vi "Read value Elevator Position.vi"(8 "error in (no error)":errorcluster, 11 "Sim Sensor Interface in":refnum<class "Sim Sensor Interface.lvclass">) -> (0 "error out":errorcluster, 3 "Sim Sensor Interface out":refnum<class "Sim Sensor Interface.lvclass">)   [LabVIEW 2019, in "Simulated Sensor Interface Actor.lvlib" / "Sim Sensor Interface.lvclass"]
uses:
  Sim Sensor Interface.lvclass
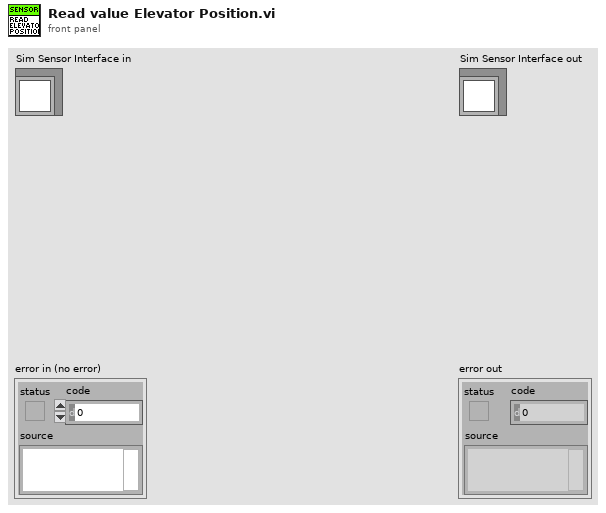
[diagram p1: front panel]
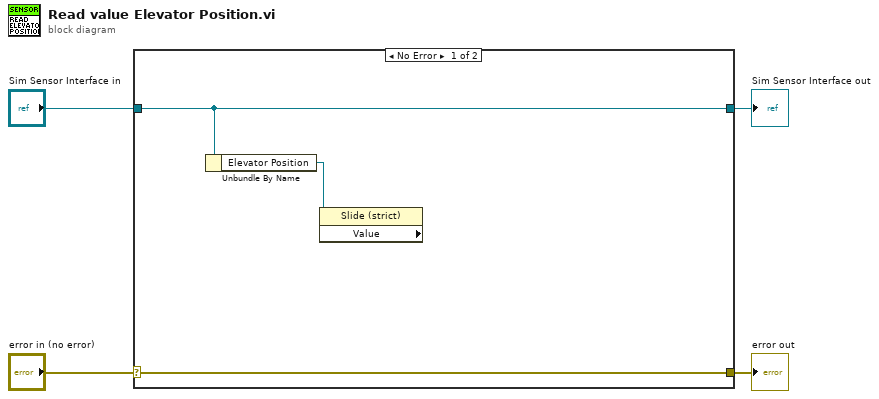
[diagram p0: block diagram]
diagram:
  n1 = case shown="No Error" "error in (no error)" {
    selector: "error in (no error)" -> [w7 w9]
    tunnel: [w7 w9] -> w3
    tunnel: [w6 w8] -> w1
    tunnel: "Sim Sensor Interface in" -> [w6 w8]
    frame No Error {
      n2 = Unbundle By Name(w6) -> ("Elevator Position"=w5:refnum<vi>)
      n3 = property class="Slide (strict)" props=["Value"](reference=w5) -> ()  [unwired: 1 in, 3 out]
    }
    frame Error {
    }
  }
  "error out" <- w3
  "Sim Sensor Interface out" <- w1
